vi "Patch data preview-Initialise montage gen.vi"(0 "ExperimentPath":path, 11 "error in (no error)":errorcluster, 13 "Number of rows to generate":i32=6) -> (3 "Experiment Parameters":T3, 4 "Image ref (Montage)":T2, 6 "Coordinates of montage positions":cluster{"X\n\nY":i32[]}[](array[cluster]), 8 "TDMS references(All Trials)":refnum<k34>[](array[refnum]), 10 "Frames info":T1, 15 "error out":errorcluster)   [LabVIEW 2017]
uses:
  User Interface/Visualisation/Patch-Vol video generator/Typedefs/Experiment Parameters.ctl
  <vilib>/vision/Image Controls.llb/IMAQ Image.ctl
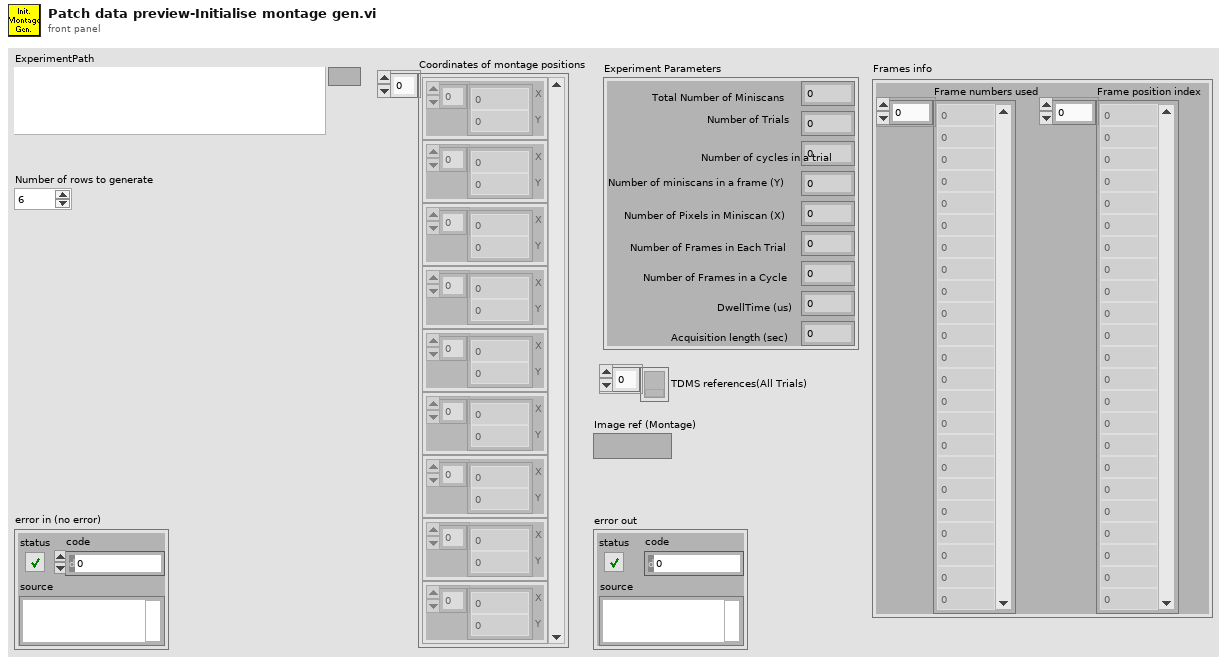
[diagram p1: front panel]
types:
  T1 = cluster{"Frame numbers used":i32[], "Frame position index":i32[]}
  T2 = typedef "IMAQ Image.ctl" = refnum<image>
  T3 = typedef "Experiment Parameters.ctl" = cluster{"Total Number of Miniscans":i32, "Number of Trials":i32, "Number of cycles in a trial":i32, "Number of miniscans in a frame (Y)":i32, "Number of Pixels in Miniscan (X)":i32, "Number of Frames in Each Trial":i32, "Number of Frames in a Cycle":i32, "DwellTime (us)":dbl, "Acquisition length (sec)":dbl}
  T4 = cluster{"Number of rows to generate":i32, "Number of columns to generate":i32}
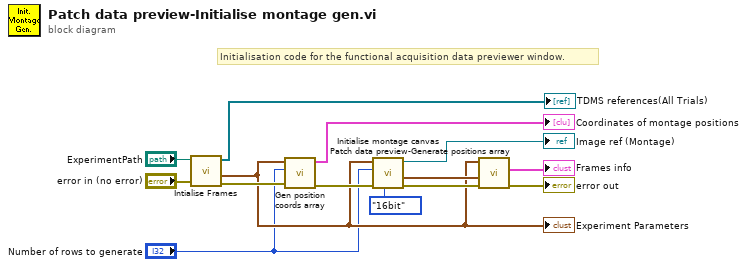
[diagram p0: block diagram]
diagram:
  # "Initialisation code for the functional acquisition data previewer window."
  n1 = call "Intialise Frames.vi"("error in (no error)"="error in (no error)", "ExperimentPath"="ExperimentPath") -> ("error out"=w13:errorcluster, "Experiment Parameters"=w5:T3, "TDMS references(All Trials)"=→"TDMS references(All Trials)":refnum<k34>[])  [unwired: 6 in, 1 out]
  "Experiment Parameters" <- w5
  n2 = call "Gen position coords array.vi"("Error in"=w13, "Number of rows to generate"="Number of rows to generate", "Experiment Parameters"=w5) -> ("error out"=w11:errorcluster, "Coordinates of montage positions"=→"Coordinates of montage positions":cluster{"X\n\nY":i32[]}[])  [unwired: 7 in]
  n3 = call "Initialise montage canvas.vi"("Image bitness"=enum16{"8bit", "16bit"}."16bit", "Error in"=w11, "Number of rows to generate"="Number of rows to generate", "Experiment Parameters"=w5) -> ("error out"=w9:errorcluster, "Rows/Columns"=w8:T4, "I16 Image ref (Montage)"=→"Image ref (Montage)":T2)  [unwired: 4 in, 1 out]
  n4 = call "Patch data preview-Generate positions array.vi"("Error in"=w9, "Rows/Columns"=w8, "Experiment Parameters"=w5) -> ("error out"=→"error out":errorcluster, "Frames info"=→"Frames info":T1)  [unwired: 7 in]
